vi "error_handler.vi"(8 "Error In":errorcluster, 10 "Reset":bool) -> (0 "Error Out":errorcluster)   [LabVIEW 2014]
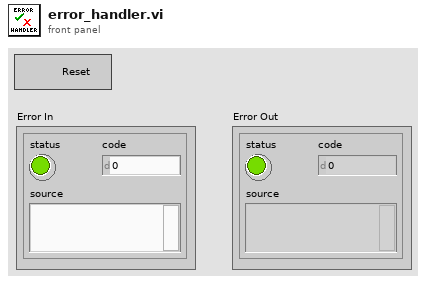
[diagram p1: front panel]
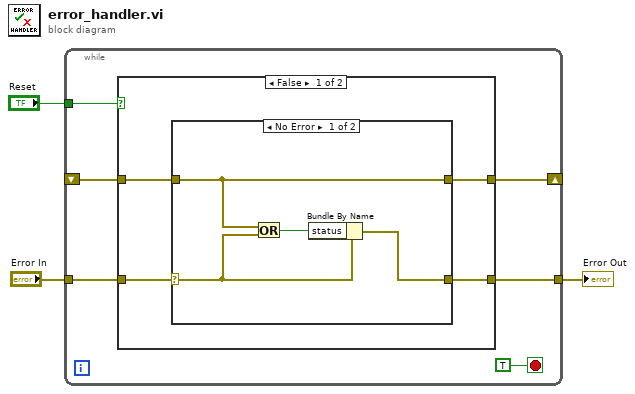
[diagram p0: block diagram]
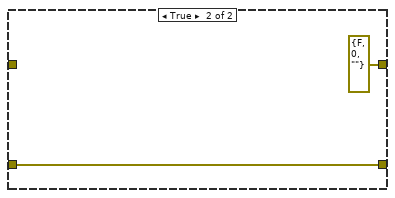
[diagram p3: hidden frame]
diagram:
  n1 = while {
    shift-right: [w6] -> _
    shift-left: _ -> [w5]
    tunnel: "Error In" -> [w8]
    tunnel: [w7] -> w2
    tunnel: "Reset" -> [w4]
    stop <- TRUE stop-if-true
    n2 = case shown="False" w4 {
      tunnel: w8 -> [w13 w19]
      tunnel: [w12 w19] -> w7
      tunnel: [w11 errorcluster {"status"=FALSE, "code"=0, "source"=""} ("error IO")] -> w6
      tunnel: w5 -> [w10 _]
      frame False {
        n3 = case shown="No Error" w13 {
          selector: w13 -> [w17 w18]
          tunnel: [w15 w18] -> w12
          tunnel: [w14 w18] -> w11
          tunnel: w10 -> [w14 _]
          frame No Error {
            n4 = Or(x=w14, y=w17) -> (x .or. y?=w16:bool)
            n5 = Bundle By Name(cluster=w17, "status"=w16) -> (w15:errorcluster)
          }
          frame Error {
          }
        }
      }
      frame True {
      }
    }
  }
  "Error Out" <- w2
